vi "JAUS Compute Target Bearing.vi"(1 "Initial Yaw In":dbl, 2 "LocalPose in":T3, 3 "Local Waypoint List Out":T1[](array[typedef])) -> (0 "Target Bearing (Yaw) (degrees)":dbl)   [LabVIEW 2009]
uses:
  JAUS/Support Files/LocalPose.ctl
  JAUS/Support Files/TimeRec.ctl
  JAUS/Support Files/ElementRec.ctl
  JAUS/Support Files/LocalWaypointRec.ctl
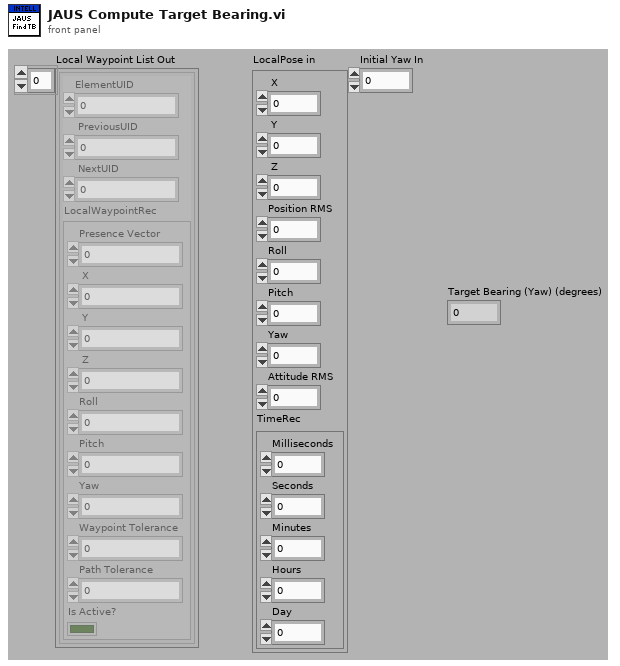
[diagram p1: front panel]
types:
  T1 = typedef "ElementRec.ctl" = cluster{"ElementUID":u16, " PreviousUID":u16, " NextUID":u16, "LocalWaypointRec":T2}
  T2 = typedef "LocalWaypointRec.ctl" = cluster{"Presence Vector":u8, " X":dbl, " Y":dbl, " Z":dbl, "Roll":dbl, "Pitch":dbl, "Yaw":dbl, "Waypoint Tolerance":dbl, "Path Tolerance":dbl, "Is Active?":bool}
  T3 = typedef "LocalPose.ctl" = cluster{" X":dbl, " Y":dbl, " Z":dbl, "Position RMS":dbl, "Roll":dbl, "Pitch":dbl, "Yaw":dbl, "Attitude RMS":dbl, "TimeRec":T4}
  T4 = typedef "TimeRec.ctl" = cluster{"Milliseconds":u32, "Seconds":u32, "Minutes":u32, "Hours":u32, "Day":u32}
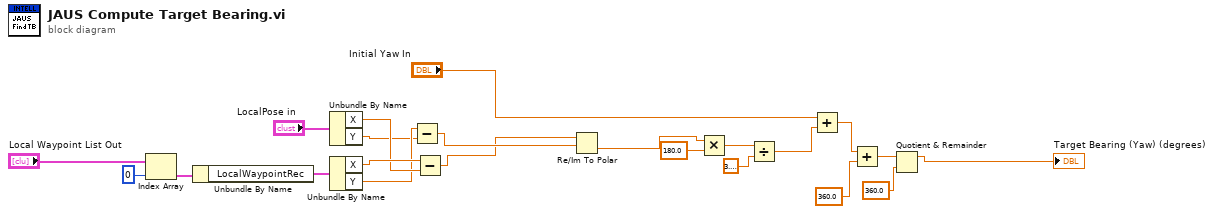
[diagram p0: block diagram]
diagram:
  n1 = Index Array(array="Local Waypoint List Out", index=0) -> (element=w20:T1)
  n2 = Unbundle By Name(w20) -> ("LocalWaypointRec"=w19:T2)
  n3 = Unbundle By Name("LocalPose in") -> ("X"=w16:dbl, "Y"=w14:dbl)
  n4 = Unbundle By Name(w19) -> ("X"=w17:dbl, "Y"=w15:dbl)
  n5 = Subtract(x=w15, y=w14) -> (x-y=w12:dbl)
  n6 = Subtract(x=w17, y=w16) -> (x-y=w11:dbl)
  n7 = Re/Im To Polar(2:w12, 3:w11) -> (0:w3:dbl)  [unwired: 1 out]
  n8 = Multiply(x=w3, y=180.0) -> (x*y=w8:dbl)
  n9 = Divide(x=w8, y=3.141592653589793) -> (x/y=w2:dbl)
  n10 = Add(x="Initial Yaw In", y=w2) -> (x+y=w1:dbl)
  n11 = Add(x=w1, y=360.0) -> (x+y=w5:dbl)
  n12 = Quotient & Remainder(x=w5, y=360.0) -> (x-y*floor(x/y)=→"Target Bearing (Yaw) (degrees)":dbl)  [unwired: 1 out]
